vi "Periodic Tasks.vi"(8 "error in":errorcluster) -> ()   [LabVIEW 2019]
doc: "This VI runs in parallel to other tasks. It can contain as many user-defined periodic loops as you need. These can carry out PID or other sorts of timed response."
uses:
  <vilib>/Rock Robotics/WPI/DriverStation/WPI_DriverStationRobotMode2.ctl
  <vilib>/Rock Robotics/WPI/Utilities/WPI_GetSetVariantRefNum.vi
  Robot Global Data.vi
  <vilib>/Rock Robotics/WPI/RobotDrive/WPI_RobotDriveArcadeDrive_Standard(NoSaturation).vi
  <vilib>/Rock Robotics/Network Tables/NT Write Numeric Array.vi
  <vilib>/Rock Robotics/Network Tables/NT Write Number.vi
  <vilib>/Rock Robotics/Network Tables/NT Write String.vi
  <vilib>/Rock Robotics/Network Tables/NT Write Boolean.vi
panel:
  in  "Yellow":cluster{"R":dbl, "G":dbl, "B":dbl}
  in  "Blue":cluster{"R":dbl, "G":dbl, "B":dbl}
  in  "Green":cluster{"R":dbl, "G":dbl, "B":dbl}
  in  "Red":cluster{"R":dbl, "G":dbl, "B":dbl}
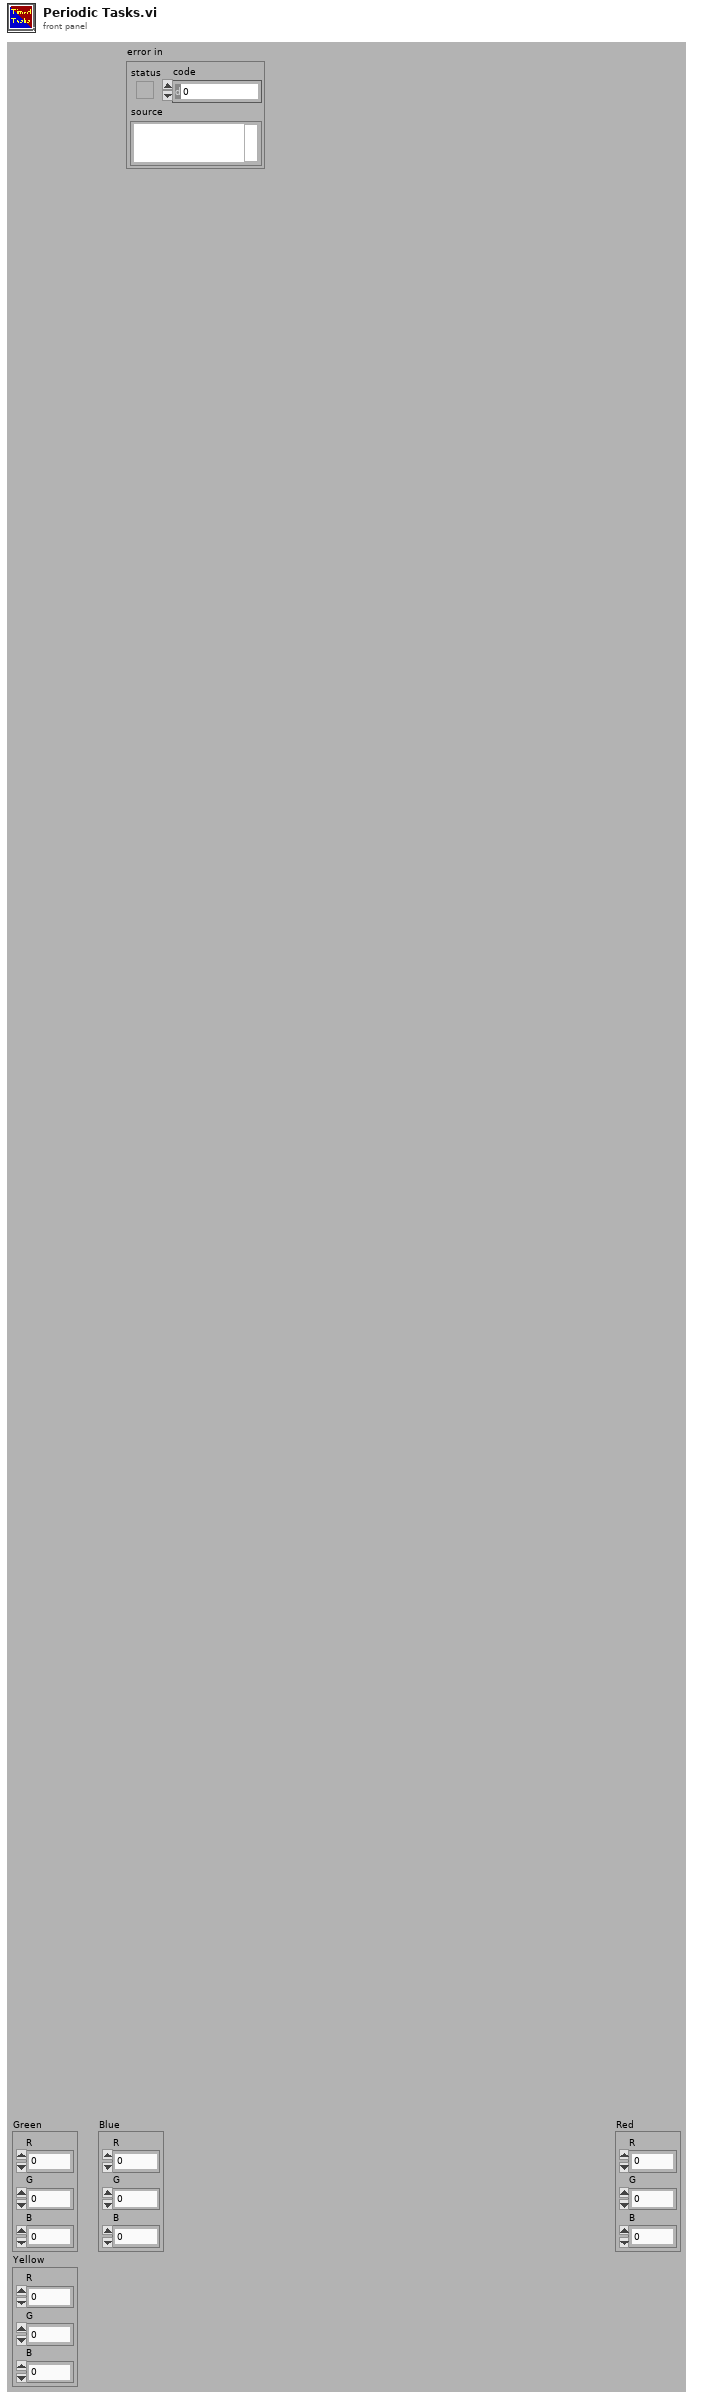
[diagram p1: front panel]
types:
  T1 = typedef "WPI_RobotDriveDevRef.ctl" = cluster{"DevStatus":errorcluster, "Motors[]":T2[], "Square Inputs":bool, "Max Output":dbl}
  T2 = typedef "WPI_MotorControlDeviceRef.ctl" = cluster{"DeviceStatus":errorcluster, "Type":T3, "PWM":cluster{"PWM Channel":T4, "DeadBand":T5}, "CAN":cluster{"Device Number":u8, "SetOutput VI Ref":variant, "GetOutput VI Ref":variant, "Enable VI Ref":variant, "Disable VI Ref":variant, "Data":variant}, "Invert":bool, "DIO PWM":cluster{"PWM \"Enable\" Channel":T4, "DIOChannel":T6, "PWM Rate":dbl}}
  T3 = typedef "WPI_MotorControlType.ctl" = enum16{"PWM", "CAN", "DIO PWM"}
  T4 = typedef "FPGA_DIOPWMChannel.ctl" = enum8{"PWM 0", "PWM 1", "PWM 2", "PWM 3", "PWM 4", "PWM 5", "PWM 6", "PWM 7", "PWM 8", "PWM 9", "PWM MXP 0", "PWM MXP 1", "PWM MXP 2", "PWM MXP 3", "PWM MXP 4", "PWM MXP 5", "PWM MXP 6", "PWM MXP 7", "PWM MXP 8", "PWM MXP 9", "Invalid"}
  T5 = typedef "WPI_PWMDeadband.ctl" = cluster{"Name":string, "maxPositivePwm":i32, "minPositivePwm":i32, "centerPwm":i32, "maxNegativePwm":i32, "minNegativePwm":i32, "angularRange":u16}
  T6 = typedef "FPGA_DIOChannel.ctl" = enum8{"DIO 0", "DIO 1", "DIO 2", "DIO 3", "DIO 4", "DIO 5", "DIO 6", "DIO 7", "DIO 8", "DIO 9", "DIO MXP 0", "DIO MXP 1", "DIO MXP 2", "DIO MXP 3", "DIO MXP 4", "DIO MXP 5", "DIO MXP 6", "DIO MXP 7", "DIO MXP 8", "DIO MXP 9", "DIO MXP 10", "DIO MXP 11", "DIO MXP 12", "DIO MXP 13", "DIO MXP 14", "DIO MXP 15", "SPI Port CS1", "SPI Port CS2", "SPI Port CS3", "SPI Port MISO", "SPI Port MOSI", "Invalid"}
  T7 = typedef "WPI_JoystickDevRef.ctl" = cluster{"Device":T8}
  T8 = typedef "WPI_JoystickDeviceEnum.ctl" = enum16{"USB 0", "USB 1", "USB 2", "USB 3", "USB 4", "USB 5"}
  T9 = cluster{"JoystickDevRef":T7, "RobotDriveDevRef":T1}
  T10 = typedef "WPI_GyroDevRef.ctl" = cluster{"DevStatus":errorcluster, "Analog Channel":T11, "Gain (VoltsPerDegree/Second)":dbl, "Gyro Type":enum16{"Analog", "XRS450"}, "Handle":i32, "SPI Bus":T12, "Device Found":bool, "Sample Rate":dbl, "Calibrate On Open":bool, "Offset":dbl}
  T11 = typedef "FPGA_AIChannel.ctl" = enum8{"AI 0", "AI 1", "AI 2", "AI 3", "AI MXP 0", "AI MXP 1", "AI MXP 2", "AI MXP 3", "Invalid"}
  T12 = typedef "spi_bus.ctl" = enum16{"SPI On-Board, CS0", "SPI On-Board, CS1", "SPI On-Board, CS2", "SPI On-Board, CS3", "SPI MXP", "Invalid"}
  T13 = typedef "WPI_DriverStationRobotMode2.ctl" = enum16{"Autonomous Disabled", "Autonomous Enabled", "Teleop Disabled", "Teleop Enabled", "Disconnected", "Finish", "Test Disabled", "Test Enabled", "Emergency Stopped"}
  T14 = typedef "Color Sensor V3 DevRef.ctl" = cluster{"I2CDevRef":T15}
  T15 = typedef "WPI_I2CDevRef.ctl" = cluster{"DevStatus":errorcluster, "Device Address":u8, "Handle":i32, "I2C Bus":T16}
  T16 = typedef "i2c_bus.ctl" = enum16{"I2C On-Board", "I2C MXP", "Invalid"}
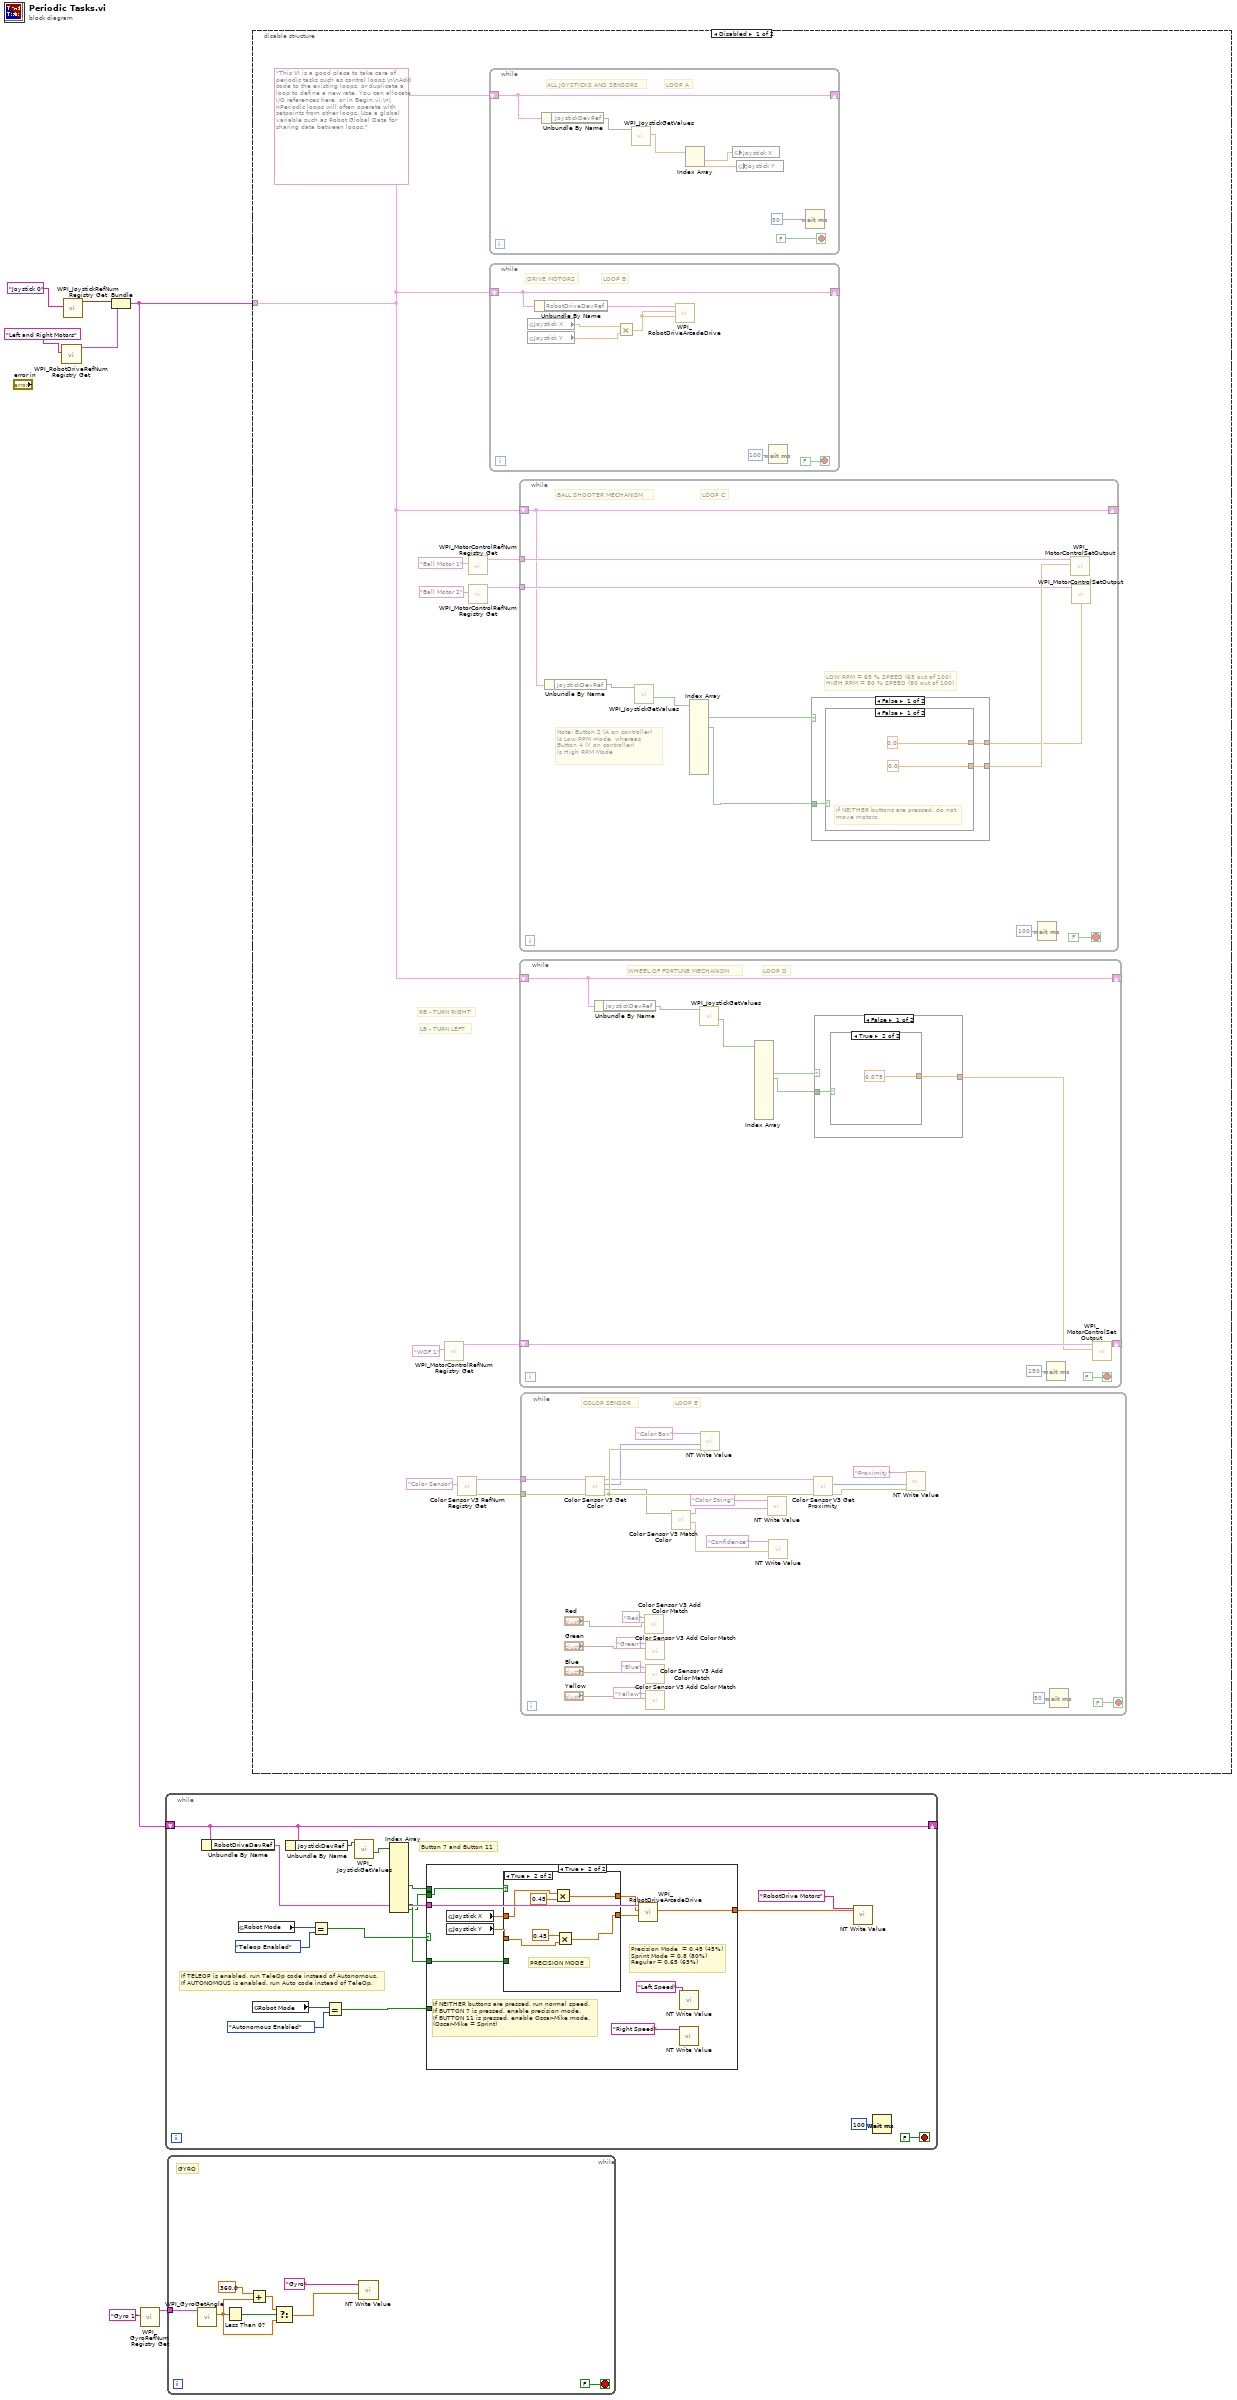
[diagram p0: block diagram]
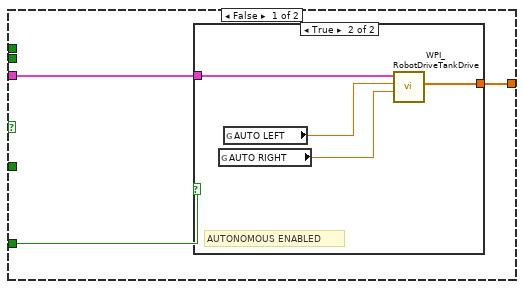
[diagram p2: hidden frame]
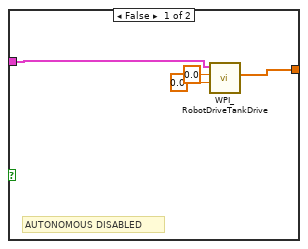
[diagram p3: hidden frame]
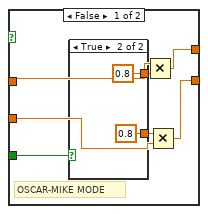
[diagram p4: hidden frame]
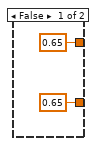
[diagram p5: hidden frame]
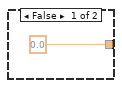
[diagram p6: hidden frame]
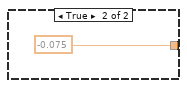
[diagram p7: hidden frame]
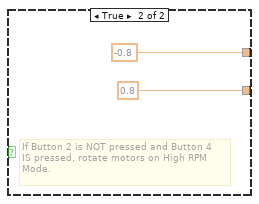
[diagram p8: hidden frame]
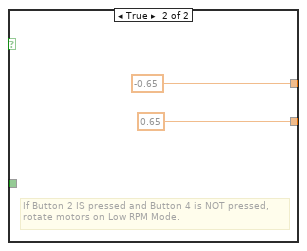
[diagram p9: hidden frame]
diagram:
  n1 = call <vilib>:"WPI_RobotDriveRefNum Registry Get.vi"("refnum name"="Left and Right Motors") -> ("RobotDriveDevRef"=w7:T1)  [unwired: 1 in, 9 out]
  n2 = call <vilib>:"WPI_JoystickRefNum Registry Get.vi"("refnum name"="Joystick 0") -> ("JoystickDevRef"=w6:T7)  [unwired: 1 in, 9 out]
  n3 = Bundle("JoystickDevRef"=w6, "RobotDriveDevRef"=w7) -> (w3:T9)  [unwired: 1 out]
  n4 = call <vilib>:"WPI_GyroRefNum Registry Get.vi"("refnum name"="Gyro 1") -> ("GyroDevRef"=w2:T10)  [unwired: 9 in, 1 out]
  n5 = while {
    shift-right: [w13] -> _
    shift-left: w3 -> [w13]
    stop <- FALSE stop-if-true
    # "Button 7 and Button 11"
    # "If TELEOP is enabled, run TeleOp code instead of Autonomous.\nIf AUTONOMOUS is enabled, run Auto code instead of TeleOp."
    n6 = Unbundle By Name(w13) -> ("RobotDriveDevRef"=w20:T1)
    n7 = global read "Robot Global Data.vi" "Robot Mode"() -> (w18:T13)
    n8 = global read "Robot Global Data.vi" "Robot Mode"() -> (w16:T13)
    n9 = Unbundle By Name(w13) -> ("JoystickDevRef"=w12:T7)
    n10 = Equal?(x=w18, y=WPI_DriverStationRobotMode2."Teleop Enabled") -> (x = y?=w19:bool)
    n11 = Equal?(x=w16, y=WPI_DriverStationRobotMode2."Autonomous Enabled") -> (x = y?=w14:bool)
    n12 = call <vilib>:"WPI_JoystickGetValues.vi"("JoystickDevRef"=w12) -> ("Buttons"=w11:bool[])  [unwired: 6 in, 4 out]
    n13 = Index Array(array=w11) -> (element #7=w10:bool, element #11=w9:bool, element #12=w8:bool)  [unwired: 12 in, 9 out]
    n14 = case shown="True" w19 {
      tunnel: [w27 w44] -> w21
      tunnel: w20 -> [w26 w45]
      tunnel: w14 -> [w25 _]
      tunnel: w10 -> [_ _]
      tunnel: w9 -> [_ w39]
      tunnel: w8 -> [_ w38]
      frame False {
        n15 = case shown="True" w25 {
          tunnel: [w31 w35] -> w27
          tunnel: w26 -> [w28 w33]
          frame False {
            # "AUTONOMOUS DISABLED"
            n16 = call <vilib>:"WPI_RobotDriveTankDrive.vi"("Right axis value"=0.0, "Left axis value"=0.0, "RobotDriveDevRef"=w28) -> ("Motor Values"=w31:dbl[])  [unwired: 6 in, 2 out]
          }
          frame True {
            # "AUTONOMOUS ENABLED"
            n17 = global read "Robot Global Data.vi" "AUTO RIGHT"() -> (w32:dbl)
            n18 = global read "Robot Global Data.vi" "AUTO LEFT"() -> (w34:dbl)
            n19 = call <vilib>:"WPI_RobotDriveTankDrive.vi"("Right axis value"=w32, "Left axis value"=w34, "RobotDriveDevRef"=w33) -> ("Motor Values"=w35:dbl[])  [unwired: 6 in, 2 out]
          }
        }
      }
      frame True {
        # "Precision Mode  = 0.45 (45%)\nSprint Mode = 0.8 (80%)\nRegular = 0.65 (65%)"
        # "If NEITHER buttons are pressed, run normal speed.\nIf BUTTON 7 is pressed, enable precision mode.\nIf BUTTON 11 is pressed, enable Oscar-Mike mode.\n(Oscar-Mike = Sprint)"
        n20 = global read "Robot Global Data.vi" "Joystick X"() -> (w43:dbl)
        n21 = global read "Robot Global Data.vi" "Joystick Y"() -> (w42:dbl)
        n22 = case shown="True" w38 {
          tunnel: w43 -> [w49 w58]
          tunnel: w42 -> [w50 w57]
          tunnel: [w48 w59] -> w41
          tunnel: [w47 w60] -> w40
          tunnel: w39 -> [w46 _]
          frame False {
            # "OSCAR-MIKE MODE"
            n23 = case shown="True" w46 {
              tunnel: [0.65 ("x") 0.8 ("x")] -> w52
              tunnel: [0.65 ("y") 0.8 ("y")] -> w51
              frame False {
              }
              frame True {
              }
            }
            n24 = Multiply(x=w49, y=w51) -> (x*y=w48:dbl)
            n25 = Multiply(x=w52, y=w50) -> (x*y=w47:dbl)
          }
          frame True {
            # "PRECISION MODE"
            n26 = Multiply(x=w58, y=0.45) -> (x*y=w59:dbl)
            n27 = Multiply(x=0.45, y=w57) -> (x*y=w60:dbl)
          }
        }
        n28 = call-poly <vilib>:"WPI_RobotDriveArcadeDrive.vi"("Y axis value"=w40, "X axis value"=w41, "RobotDriveDevRef"=w45) -> ("Motor Values"=w44:dbl[])  [unwired: 6 in, 2 out]
        n29 = call-poly <vilib>:"NT Write Value.vi"("Name"="Right Speed") -> ()  [unwired: 10 in, 1 out]
        n30 = call-poly <vilib>:"NT Write Value.vi"("Name"="Left Speed") -> ()  [unwired: 10 in, 1 out]
      }
    }
    n31 = call-poly <vilib>:"NT Write Value.vi"("Numeric Array"=w21, "Name"="RobotDrive Motors") -> ()  [unwired: 9 in, 1 out]
    n32 = Wait (ms)(milliseconds to wait=u32 100) -> ()  [unwired: 1 out]
  }
  n33 = while {
    tunnel: w2 -> [w69]
    stop <- FALSE stop-if-true
    # "GYRO"
    n34 = call <vilib>:"WPI_GyroGetAngle.vi"("GyroDevRef"=w69) -> ("Angle"=w65:dbl)  [unwired: 6 in, 4 out]
    n35 = Less Than 0?(x=w65) -> (x < 0?=w68:bool)
    n36 = Add(x=360.0, y=w65) -> (x+y=w66:dbl)
    n37 = Select(t=w66, s=w68, f=w65) -> (s? t:f=w64:dbl)
    n38 = call-poly <vilib>:"NT Write Value.vi"("Numeric"=w64, "Name"="Gyro") -> ()  [unwired: 9 in, 1 out]
  }
  n39 = disable-structure shown="Disabled" {
    disable-tunnel: w3 -> [w71 _]
    frame Disabled {
      (unwired) "This VI is a good place to take care of periodic tasks such as control loops.\n\nAdd code to the existing loops, or duplicate a loop to define a new rate. You can allocate I/O references here, or in Begin.vi.\n\nPeriodic loops will often operate with setpoints from other loops. Use a global variable such as Robot Global Data for sharing data between loops."
      # "LB - TURN LEFT"
      # "RB - TURN RIGHT"
      n40 = call <vilib>:"WPI_MotorControlRefNum Registry Get.vi"("refnum name"="WOF 1") -> ("MotorControlDevRef"=w75:T2)  [unwired: 9 in, 1 out]
      n41 = call <vilib>:"Color Sensor V3 RefNum Registry Get.vi"("refnum name"="Color Sensor") -> ("error out"=w72:errorcluster, "ColorSensorDevRef"=w74:T14)  [unwired: 9 in]
      n42 = call <vilib>:"WPI_MotorControlRefNum Registry Get.vi"("refnum name"="Ball Motor 1") -> ("MotorControlDevRef"=w78:T2)  [unwired: 9 in, 1 out]
      n43 = call <vilib>:"WPI_MotorControlRefNum Registry Get.vi"("refnum name"="Ball Motor 2") -> ("MotorControlDevRef"=w77:T2)  [unwired: 9 in, 1 out]
      n44 = while {
        shift-right: [w152] -> _
        shift-left: w71 -> [w152]
        stop <- FALSE stop-if-true
        # "LOOP A"
        # "ALL JOYSTICKS AND SENSORS"
        n45 = Unbundle By Name(w152) -> ("JoystickDevRef"=w151:T7)
        n46 = call <vilib>:"WPI_JoystickGetValues.vi"("JoystickDevRef"=w151) -> ("Axes"=w150:dbl[])  [unwired: 6 in, 4 out]
        n47 = Index Array(array=w150) -> (element #1=w148:dbl, element #2=w149:dbl)  [unwired: 2 in]
        n48 = global write "Robot Global Data.vi" "Joystick X"(w148) -> ()
        n49 = global write "Robot Global Data.vi" "Joystick Y"(w149) -> ()
        n50 = Wait (ms)(milliseconds to wait=u32 50) -> ()  [unwired: 1 out]
      }
      n51 = while {
        shift-right: [w144] -> _
        shift-left: w71 -> [w144]
        stop <- FALSE stop-if-true
        # "LOOP B"
        # "DRIVE MOTORS"
        n52 = global read "Robot Global Data.vi" "Joystick X"() -> (w140:dbl)
        n53 = global read "Robot Global Data.vi" "Joystick Y"() -> (w141:dbl)
        n54 = Unbundle By Name(w144) -> ("RobotDriveDevRef"=w143:T1)
        n55 = Multiply(x=w140, y=w141) -> (x*y=w142:dbl)
        n56 = call-poly <vilib>:"WPI_RobotDriveArcadeDrive.vi"("Y axis value"=w142, "X axis value"=w142, "RobotDriveDevRef"=w143) -> ()  [unwired: 6 in, 3 out]
        n57 = Wait (ms)(milliseconds to wait=u32 100) -> ()  [unwired: 1 out]
      }
      n58 = while {
        shift-right: [w124] -> _
        shift-left: w71 -> [w124]
        tunnel: w78 -> [w128]
        tunnel: w77 -> [w125]
        stop <- FALSE stop-if-true
        # "LOW RPM = 65 % SPEED (65 out of 100)\nHIGH RPM = 80 % SPEED (80 out of 100)"
        # "LOOP C"
        # "Note: Button 2 (A on controller) \nis Low RPM mode, whereas \nButton 4 (Y on controller)\nis High RPM Mode"
        # "BALL SHOOTER MECHANISM"
        n59 = Unbundle By Name(w124) -> ("JoystickDevRef"=w123:T7)
        n60 = call <vilib>:"WPI_JoystickGetValues.vi"("JoystickDevRef"=w123) -> ("Buttons"=w122:bool[])  [unwired: 6 in, 4 out]
        n61 = Index Array(array=w122) -> (element #2=w120:bool, element #4=w121:bool)  [unwired: 13 in, 11 out]
        n62 = case shown="False" w120 {
          tunnel: [w133 0.65 ("Output")] -> w127
          tunnel: [w132 -0.65 ("Output")] -> w126
          tunnel: w121 -> [w131 _]
          frame False {
            n63 = case shown="False" w131 {
              tunnel: [0.0 ("Output") 0.8 ("Output")] -> w133
              tunnel: [0.0 ("Output") -0.8 ("Output")] -> w132
              frame False {
                # "If NEITHER buttons are pressed, do not\nmove motors."
              }
              frame True {
                # "If Button 2 is NOT pressed and Button 4\nIS pressed, rotate motors on High RPM\nMode."
              }
            }
          }
          frame True {
            # "If Button 2 IS pressed and Button 4 is NOT pressed,\nrotate motors on Low RPM Mode."
          }
        }
        n64 = Wait (ms)(milliseconds to wait=u32 100) -> ()  [unwired: 1 out]
        n65 = call <vilib>:"WPI_MotorControlSetOutput.vi"("Output"=w127, "MotorControlDevRef"=w128) -> ()  [unwired: 7 in, 3 out]
        n66 = call <vilib>:"WPI_MotorControlSetOutput.vi"("Output"=w126, "MotorControlDevRef"=w125) -> ()  [unwired: 7 in, 3 out]
      }
      n67 = while {
        shift-right: [w113] -> _
        shift-left: w71 -> [w113]
        shift-right: [w109] -> _
        shift-left: w75 -> [w110]
        stop <- FALSE stop-if-true
        # "LOOP D"
        # "WHEEL OF FORTUNE MECHANISM"
        n68 = Unbundle By Name(w113) -> ("JoystickDevRef"=w112:T7)
        n69 = call <vilib>:"WPI_JoystickGetValues.vi"("JoystickDevRef"=w112) -> ("Buttons"=w111:bool[])  [unwired: 6 in, 4 out]
        n70 = Index Array(array=w111) -> (element #5=w107:bool, element #6=w106:bool)  [unwired: 14 in, 12 out]
        n71 = case shown="False" w107 {
          tunnel: [w115 -0.075 ("Output")] -> w108
          tunnel: w106 -> [w116 _]
          frame False {
            n72 = case shown="True" w116 {
              tunnel: [0.0 ("Output") 0.075 ("Output")] -> w115
              frame False {
              }
              frame True {
              }
            }
          }
          frame True {
          }
        }
        n73 = Wait (ms)(milliseconds to wait=u32 150) -> ()  [unwired: 1 out]
        n74 = call <vilib>:"WPI_MotorControlSetOutput.vi"("Output"=w108, "MotorControlDevRef"=w110) -> ("MotorControlDevRef"=w109:T2)  [unwired: 7 in, 2 out]
      }
      n75 = while {
        tunnel: w74 -> [w103]
        tunnel: w72 -> [w102]
        stop <- FALSE stop-if-true
        # "LOOP E"
        # "COLOR SENSOR"
        n76 = call <vilib>:"Color Sensor V3 Get Color.vi"("error in (no error)"=w102, "ColorSensorDevRef"=w103) -> ("error out"=w101:errorcluster, "Normalized Color"=w95:cluster{"R":dbl, "G":dbl, "B":dbl}, "Color"=w98:u32, "ColorSensorDevRef out"=w99:T14)  [unwired: 6 in]
        n77 = call <vilib>:"Color Sensor V3 Add Color Match.vi"("Color"="Red", "Name"="Red") -> ()  [unwired: 10 in]
        n78 = call <vilib>:"Color Sensor V3 Add Color Match.vi"("Color"="Green", "Name"="Green") -> ()  [unwired: 10 in]
        n79 = call <vilib>:"Color Sensor V3 Add Color Match.vi"("Color"="Blue", "Name"="Blue") -> ()  [unwired: 10 in]
        n80 = call <vilib>:"Color Sensor V3 Add Color Match.vi"("Color"="Yellow", "Name"="Yellow") -> ()  [unwired: 10 in]
        n81 = call <vilib>:"Color Sensor V3 Match Color.vi"("Measured Color"=w95) -> ("Confidence"=w94:dbl, "Matched Color Name"=w93:string)  [unwired: 8 in, 1 out]
        n82 = call-poly <vilib>:"NT Write Value.vi"("error in"=w101, "Numeric"=w98, "Name"="Color Box") -> ()  [unwired: 8 in, 1 out]
        n83 = call-poly <vilib>:"NT Write Value.vi"("String"=w93, "Name"="Color String") -> ()  [unwired: 9 in, 1 out]
        n84 = call-poly <vilib>:"NT Write Value.vi"("Numeric"=w94, "Name"="Confidence") -> ()  [unwired: 9 in, 1 out]
        n85 = call <vilib>:"Color Sensor V3 Get Proximity.vi"("error in (no error)"=w101, "ColorSensorDevRef"=w99) -> ("error out"=w96:errorcluster, "Proximity"=w97:u16)  [unwired: 7 in, 1 out]
        n86 = call-poly <vilib>:"NT Write Value.vi"("error in"=w96, "Numeric"=w97, "Name"="Proximity") -> ()  [unwired: 8 in, 1 out]
        n87 = Wait (ms)(milliseconds to wait=u32 50) -> ()  [unwired: 1 out]
      }
    }
    frame Enabled {
    }
  }
